vi "Script Definition.vi"(4 "Project Ref":refnum<vi>, 5 "Type Path Map":map{path, path}(c390), 6 "Names":string[](array[string]), 7 "Entity Paths":T1, 8 "error in (no error)":errorcluster, 11 "Updated Definition":refnum<class "Type.lvclass">[](array[class])) -> (0 "error":errorcluster)   [LabVIEW 2020, in "Conditum-Tools.lvlib" / "Entity Editor.lvclass"]
uses:
  Entity Editor.lvclass
  Conditum-Clone/Columns/Type/Type.lvclass
  Entity Paths.ctl
  <vilib>/IlluminatedG/IG Conditum Base/Conditum/Columns/Type/Type.lvclass
  <vilib>/Utility/miscctls.llb/LVPointTypeDef.ctl
  <vilib>/_script/New VI Object TypeDefs/NewVIObject_LVRelativePositionTypeDef.ctl
  <vilib>/_script/New VI Object TypeDefs/NewVIObject_LVRelativeDirectionTypeDef.ctl
  <vilib>/Utility/miscctls.llb/LVPoint32TypeDef.ctl
  9905195a-609c-4328-ab75-e7799d536e83.vi
  <vilib>/Utility/LVClass/Get LV Class Name.vi
  <vilib>/Utility/error.llb/Error Cluster From Error Code.vi
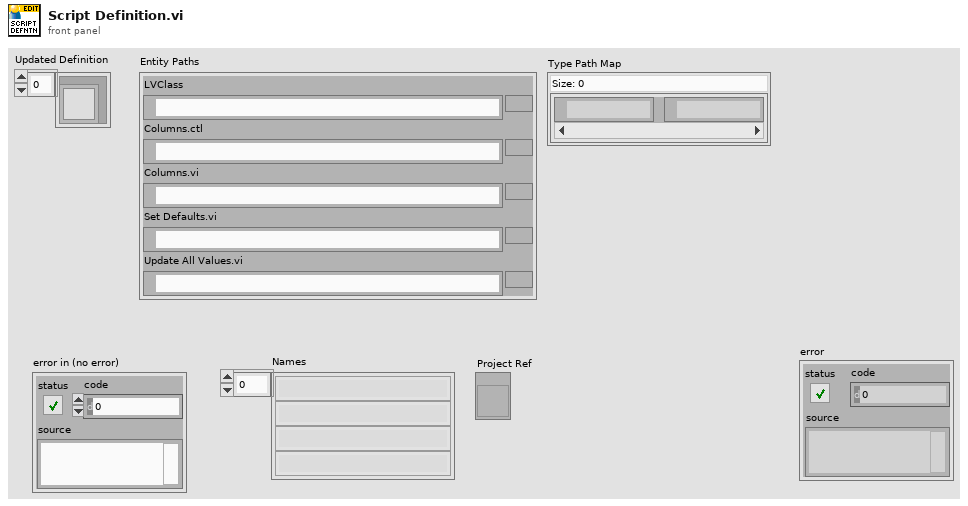
[diagram p1: front panel]
types:
  T1 = typedef "Conditum-Tools.lvlib/Entity Editor.lvclass/Entity Paths.ctl" = cluster{"LVClass":path, "Columns.ctl":path, "Columns.vi":path, "Set Defaults.vi":path, "Update All Values.vi":path}
  T2 = typedef "NewVIObject_LVRelativePositionTypeDef.ctl" = cluster{"Refnum":refnum<vi>, "Relative Direction":T3, "Point32":T4}
  T3 = typedef "NewVIObject_LVRelativeDirectionTypeDef.ctl" = enum32{"Right", "Left", "Top", "Bottom", "Top Right", "Top Left", "Bottom Right", "Bottom Left"}
  T4 = typedef "LVPoint32TypeDef.ctl" = cluster{"Horizontal":i32, "Vertical":i32}
  T5 = typedef "LVPointTypeDef.ctl" = cluster{"Horizontal":i16, "Vertical":i16}
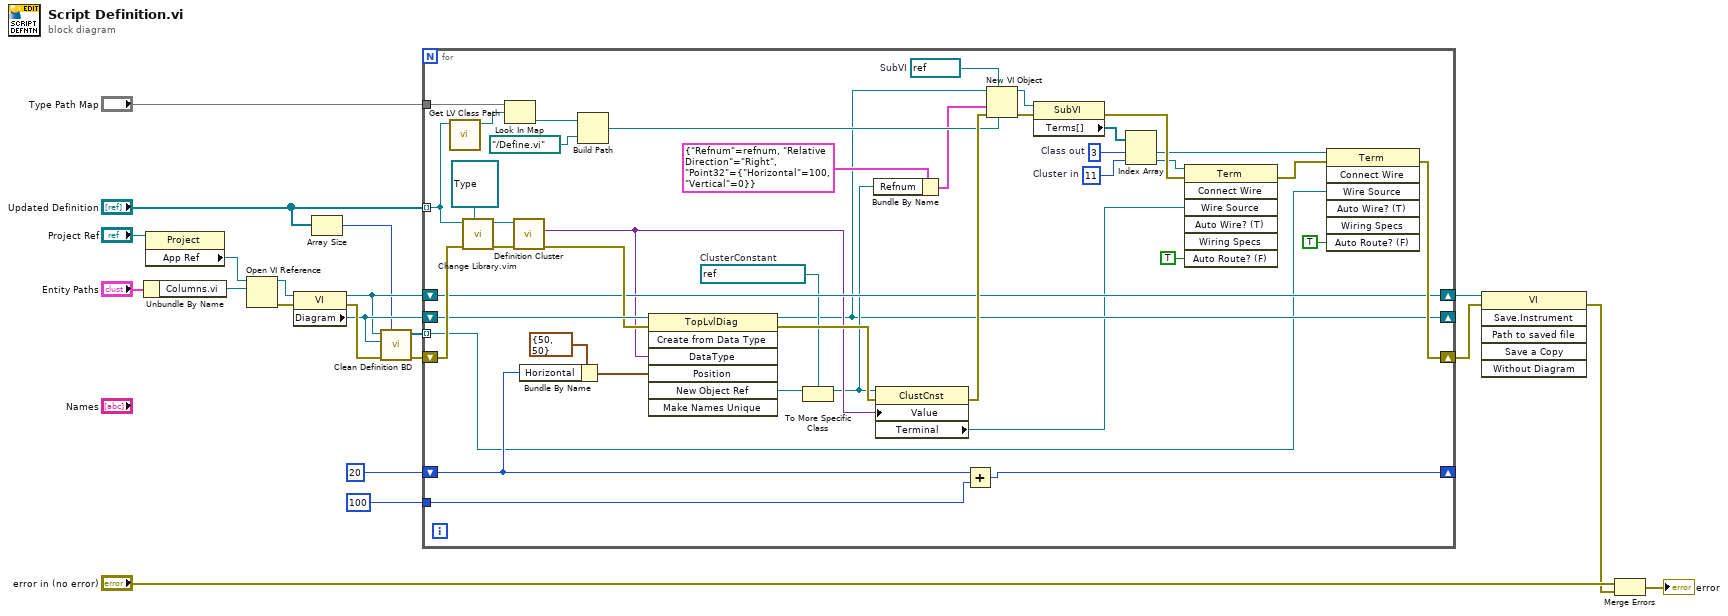
[diagram p0: block diagram]
diagram:
  n1 = Unbundle By Name("Entity Paths") -> ("Columns.vi"=w18:path)
  n2 = property class="Project"(reference="Project Ref") -> ("App Ref"=w17:refnum<vi>)  [unwired: 1 in, 2 out]
  n3 = Open VI Reference(application reference (local)=w17, vi path=w18) -> (vi reference=w15:refnum<vi>, error out=w16:errorcluster)  [unwired: 4 in]
  n4 = property class="VI"(reference=w15, error in=w16) -> (reference out=w10:refnum<vi>, error out=w21:errorcluster, "Diagram"=w11:refnum<vi>)
  n5 = Array Size(array="Updated Definition") -> (size(s)=w4:i32)
  n6 = call "Clean Definition BD.vi"("Count"=w4, "error in (no error)"=w21, "Diagram"=w11, "VI"=w10) -> ("error out"=w12:errorcluster, "Bundle Terminals"=w6:refnum<vi>[])  [unwired: 6 in]
  n7 = for {
    shift-right: [w62] -> w2
    shift-left: w12 -> [w52]
    shift-right: [w43] -> w3
    shift-left: w10 -> [w43]
    shift-right: [w35] -> _
    shift-left: w11 -> [w48]
    tunnel: "Updated Definition" -> [w54] mode=indexing
    tunnel: "Type Path Map" -> [w58]
    shift-right: [w49] -> _
    shift-left: 20 -> [w45]
    tunnel: 100 -> [w50]
    tunnel: w6 -> [w24] mode=indexing
    w29 = 11  # Cluster in
    w30 = 3  # Class out
    w34 = refnum<vi> refnum  # SubVI
    w41 = refnum<vi> refnum  # ClusterConstant
    n8 = call <vilib>:"Get LV Class Path.vi"("object"=w54) -> ("class path"=w57:path)  [unwired: 9 in, 1 out]
    n9 = call "Change Library.vim"("To Type"=refnum<class "Type.lvclass"> refnum ("Conditum:Columns:Type.lvclass"), "error in (no error)"=w52, "From Value"=w54) -> ("error out"=w44:errorcluster, "To Value"=w51:refnum<class "Type.lvclass">)  [unwired: 6 in, 1 out]
    n10 = Look In Map(map=w58, key=w57) -> (value=w56:path)  [unwired: 1 in, 1 out]
    n11 = call-dynamic "Definition Cluster.vi"("Type in"=w51) -> ("Definition"=w40:variant)  [unwired: 9 in, 1 out]
    n12 = Bundle By Name(cluster=T5 {"Horizontal"=50, "Vertical"=50} ("Position"), "Horizontal"=w45) -> (w46:T5)
    n13 = Build Path(base path=w56, name or relative path=path "../Define.vi") -> (appended path=w37:path)
    n14 = invoke class="TopLvlDiag" method="Create from Data Type"(reference=w48, error in=w44, "DataType"=w40, "Position"=w46) -> (reference out=w35:refnum<vi>, error out=w59:errorcluster, "New Object Ref"=w42:refnum<vi>)  [unwired: 3 in, 4 out]
    n15 = To More Specific Class(target class=w41, reference=w42) -> (specific class reference=w38:refnum<vi>)  [unwired: 1 in, 1 out]
    n16 = Bundle By Name(cluster=T2 {"Refnum"=refnum, "Relative Direction"=enum."Right", "Point32"={"Horizontal"=100, "Vertical"=0}} ("Relative Position"), "Refnum"=w38) -> (w36:T2)
    n17 = property class="ClustCnst"(reference=w38, error in=w59, "Value"=w40) -> (error out=w60:errorcluster, "Terminal"=w27:refnum<vi>)  [unwired: 1 out]
    n18 = Add(x=w45, y=w50) -> (x+y=w49:i32)
    n19 = New VI Object(vi object class=w34, owner refnum=w35, position/next to=w36, 6:w37, 8:w60) -> (object refnum=w33:refnum<vi>, 0:w32:errorcluster)  [unwired: 3 in]
    n20 = property class="SubVI"(reference=w33, error in=w32) -> (error out=w61:errorcluster, "Terms[]"=w31:refnum<vi>[])  [unwired: 1 out]
    n21 = Index Array(array=w31, index #1=w30, index #2=w29) -> (element #1=w25:refnum<vi>, element #2=w28:refnum<vi>)
    n22 = invoke class="Term" method="Connect Wire"(reference=w28, error in=w61, "Wire Source"=w27, "Auto Route? (F)"=TRUE) -> (error out=w22:errorcluster)  [unwired: 3 in, 6 out]
    n23 = invoke class="Term" method="Connect Wire"(reference=w25, error in=w22, "Wire Source"=w24, "Auto Route? (F)"=TRUE) -> (error out=w62:errorcluster)  [unwired: 3 in, 6 out]
  }
  n24 = invoke class="VI" method="Save.Instrument"(reference=w3, error in=w2) -> (error out=w1:errorcluster)  [unwired: 4 in, 5 out]
  n25 = Merge Errors("error in (no error)", w1) -> (→"error":errorcluster)
